vi "configure piezo and pockelscontrol for galvo.vi"() -> (0 "error out":errorcluster, 3 "task out":refnum<k21>)   [LabVIEW 2012]
uses:
  <vilib>/DAQmx/write.llb/DAQmx Write (Analog 2D DBL NChan NSamp).vi
  GFG/GFGstringGet.vi
  GFG/GFGfpRefGet.vi
  GFG/GFGnumericGet.vi
  GFG/GFGbooleanGet.vi
  <vilib>/DAQmx/create/channels.llb/DAQmx Create Channel (AO-Voltage-Basic).vi
  <vilib>/DAQmx/miscellaneous.llb/DAQmx Fill In Error Info.vi
  GFG/GFG library.lvlib
  <resource>/objmgr/daqmx.rc
panel:
  out "pockels cell control":dbl[](graph)
  out "piezo control":dbl[](graph)
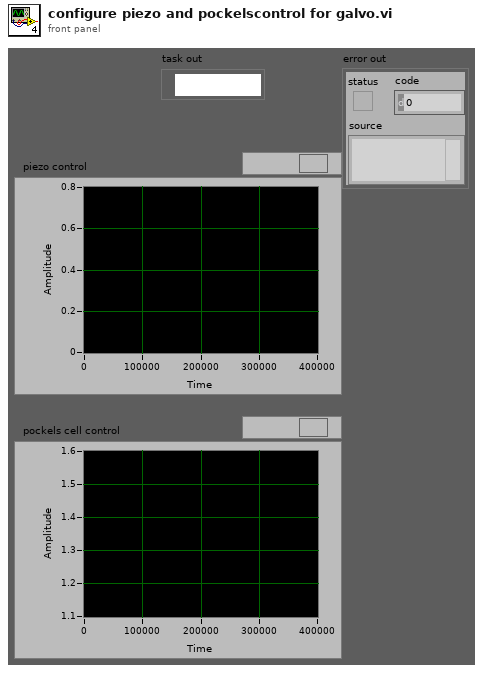
[diagram p1: front panel]
types:
  T1 = enum8{"Enabled", "Disabled", "Disabled and Grayed Out"}
  T2 = cluster{"WaveformChartRef":refnum<vi>, "DigitalRef":refnum<vi>, "ArrayRef":refnum<vi>, "TabControlRef":refnum<vi>, "EnumRef":refnum<vi>, "RingRef":refnum<vi>, "BooleanRef":refnum<vi>, "KnobRef":refnum<vi>, "SlideRef":refnum<vi>, "PathRef":refnum<vi>, "StringRef":refnum<vi>, "ComboBox":refnum<vi>, "WaveformGraphRef":refnum<vi>}
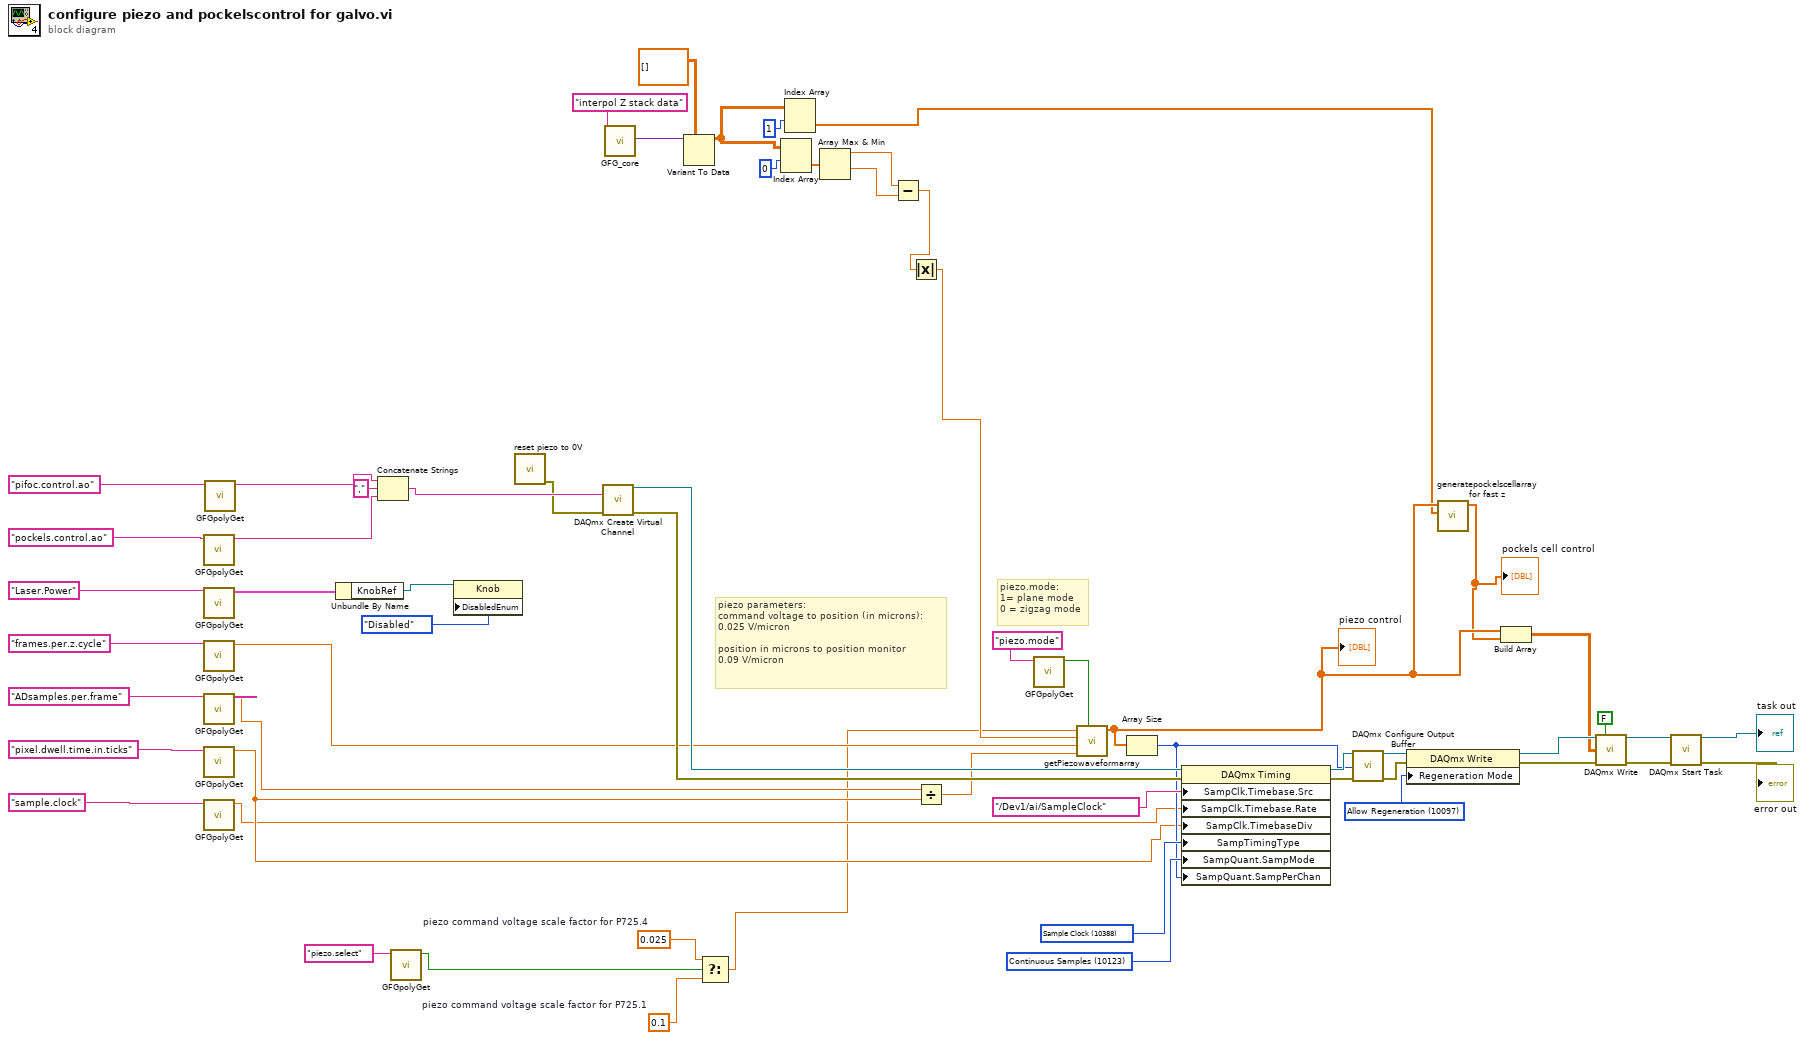
[diagram p0: block diagram]
diagram:
  w4 = 0.1  # piezo command voltage scale factor for P725.1
  w5 = 0.025  # piezo command voltage scale factor for P725.4
  w42 = 10388 items=["Sample Clock"=10388, "Burst Handshake"=12548, "Handshake"=10389, "Implicit"=10451, "On Demand"=10390, "Change Detection"=12504, "Pipelined Sample Clock"=14668] ("SampTimingType")
  w50 = 10097 items=["Allow Regeneration"=10097, "Do Not Allow Regeneration"=10158] ("RegenMode")
  w41 = 10123 items=["Finite Samples"=10178, "Continuous Samples"=10123] ("sample mode")
  # "piezo.mode: \n1= plane mode\n0 = zigzag mode"
  # "piezo parameters:\ncommand voltage to position (in microns):\n0.025 V/micron\n\nposition in microns to position monitor\n0.09 V/micron"
  n1 = call-poly "GFGpolyGet.vi"("Variable Name in"="pockels.control.ao" ("Tag in")) -> ("String"=w56:string)  [unwired: 10 in]
  n2 = call-poly "GFGpolyGet.vi"("Variable Name in"="Laser.Power") -> ("output cluster"=w54:T2)  [unwired: 9 in, 1 out]
  n3 = call-poly "GFGpolyGet.vi"("Variable Name in"="frames.per.z.cycle" ("Tag in")) -> ("Numeric"=w27:dbl)  [unwired: 9 in, 1 out]
  n4 = call-poly "GFGpolyGet.vi"("Variable Name in"="ADsamples.per.frame" ("Tag in")) -> ("Numeric"=w29:dbl)  [unwired: 9 in, 1 out]
  n5 = call-poly "GFGpolyGet.vi"("Variable Name in"="pixel.dwell.time.in.ticks" ("Tag in")) -> ("Numeric"=w31:dbl)  [unwired: 9 in, 1 out]
  n6 = call-poly "GFGpolyGet.vi"("Variable Name in"="sample.clock" ("Tag in")) -> ("Numeric"=w9:dbl)  [unwired: 9 in, 1 out]
  n7 = call-poly "GFGpolyGet.vi"("Variable Name in"="pifoc.control.ao") -> ("String"=w57:string)  [unwired: 10 in]
  n8 = Unbundle By Name(w54) -> ("KnobRef"=w53:refnum<vi>)
  n9 = Concatenate Strings(w57, "," ("string"), w56) -> (w33:string)
  n10 = call-poly "GFGpolyGet.vi"("Variable Name in"="piezo.select") -> ("Boolean"=w2:bool)  [unwired: 10 in]
  n11 = property class="Knob"(reference=w53, "DisabledEnum"=T1."Disabled" ("Disabled")) -> ()  [unwired: 1 in, 2 out]
  n12 = call "reset piezo to 0V.vi"() -> ("error out"=w8:errorcluster)  [unwired: 11 in]
  n13 = call-poly <vilib>:"DAQmx Create Virtual Channel.vi"("physical channels"=w33, "error in"=w8) -> ("task out"=w43:refnum<k21>, "error out"=w45:errorcluster)  [unwired: 12 in]
  n14 = call "GFG_core.vi"("Variable Name in"="interpol Z stack data") -> ("Variant Out"=w25:variant)  [unwired: 12 in, 6 out]
  n15 = Variant To Data(type=dbl[][] [] ("Interpolated Data"), Variant=w25) -> (data=w23:dbl[][])  [unwired: 1 in, 1 out]
  n16 = Select(t=w5, s=w2, f=w4) -> (s? t:f=w1:dbl)
  n17 = Index Array(array=w23, index (row)=0 ("disabled index (col)")) -> (element=w22:dbl[])  [unwired: 1 in]
  n18 = Index Array(array=w23, index (row)=1 ("disabled index (col)")) -> (element=w12:dbl[])  [unwired: 1 in]
  n19 = Array Max & Min(array=w22) -> (max value=w21:dbl, min value=w20:dbl)  [unwired: 2 out]
  n20 = Subtract(x=w21, y=w20) -> (x-y=w19:dbl)
  n21 = Absolute Value(x=w19) -> (abs(x)=w14:dbl)
  n22 = Divide(x=w29, y=w31) -> (x/y=w36:dbl)
  n23 = call-poly "GFGpolyGet.vi"("Variable Name in"="piezo.mode" ("Tag in")) -> ("Boolean"=w15:bool)  [unwired: 10 in]
  n24 = call "getPiezowaveformarray.vi"("planes or zigzag"=w15, "pixel.num"=w36, "frames.per.z.cycle"=w27, "total.z.distance"=w14, "piezo scale factor"=w1) -> ("Array"=w13:dbl[])  [unwired: 6 in]
  "piezo control" <- w13
  n25 = Array Size(array=w13) -> (size(s)=w35:i32)
  n26 = property class="DAQmx Timing"(reference=w43, error in=w45, "SampClk.Timebase.Src"=tag "/Dev1/ai/SampleClock" ("Clock Source"), "SampClk.Timebase.Rate"=w9, "SampClk.TimebaseDiv"=w31, "SampTimingType"=w42, "SampQuant.SampMode"=w41, "SampQuant.SampPerChan"=w35) -> (reference out=w39:refnum<k21>, error out=w46:errorcluster)
  n27 = call <vilib>:"DAQmx Configure Output Buffer.vi"("task/channels in"=w39, "buffer size (in samples per channel)"=w35, "error in"=w46) -> ("task out"=w51:refnum<k21>, "error out"=w49:errorcluster)  [unwired: 11 in]
  n28 = property class="DAQmx Write"(reference=w51, error in=w49, "Regeneration Mode"=w50) -> (reference out=w47:refnum<k21>, error out=w48:errorcluster)
  n29 = call "generatepockelscellarray for fast z.vi"("interpolated pockels cell data"=w12, "piezo control"=w13) -> ("pockelscellarray"=w11:dbl[])  [unwired: 9 in]
  "pockels cell control" <- w11
  n30 = Build Array(w13, w11) -> (w34:dbl[][])
  n31 = call-poly <vilib>:"DAQmx Write.vi"("task/channels in"=w47, "auto start"=FALSE, "data"=w34, "error in"=w48) -> ("task out"=w38:refnum<k21>, "error out"=w40:errorcluster)  [unwired: 9 in, 1 out]
  n32 = call <vilib>:"DAQmx Start Task.vi"("task/channels in"=w38, "error in"=w40) -> ("task out"=→"task out":refnum<k21>, "error out"=→"error out":errorcluster)  [unwired: 12 in]
